vi "Game_SetPlayerCash.vi"(8 "error in (no error)":errorcluster, 9 "Amount":dbl, 10 "player":T2, 11 "Players array":T1[](array[typedef])) -> (0 "error out":errorcluster, 3 "Players array OUT":T1[](array[typedef]))   [LabVIEW 2020]
uses:
  Typedefs/game_player.ctl
  Typedefs/enumeratedPlayers.ctl
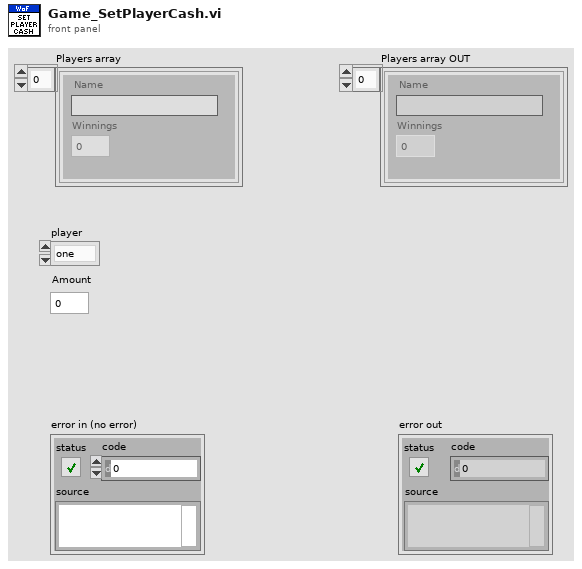
[diagram p1: front panel]
types:
  T1 = typedef "game_player.ctl" = cluster{"Name":string, "Winnings":dbl}
  T2 = typedef "enumeratedPlayers.ctl" = enum16{"one", "two", "three"}
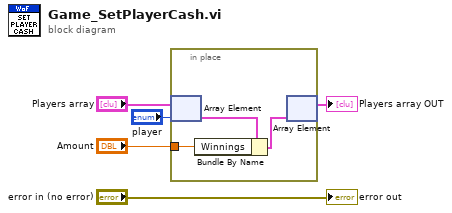
[diagram p0: block diagram]
diagram:
  n1 = in-place {
    in-place-border: "Amount" -> [w7]
    n2 = in-place-array #1("Players array", "player") -> (w8:T1)
    n3 = Bundle By Name(cluster=w8, "Winnings"=w7) -> (w6:T1)
    n4 = in-place-array #1(w6) -> (→"Players array OUT":T1[])  [unwired: 1 out]
  }
  "error out" <- "error in (no error)"
